vi "Undistort.vi"   [LabVIEW 2020, in "g_ar_toolkit.image.lvlib"]
uses:
  g_ar_toolkit.image.lvlib
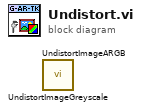
[diagram p0: block diagram]
diagram:
  n1 = call "UndistortImageGreyscale.vi"() -> ()  [unwired: 10 in, 2 out]
  n2 = call "UndistortImageARGB.vi"() -> ()  [unwired: 10 in, 2 out]
